vi "Fit Result to String.vi"(8 "error in (no error)":errorcluster, 11 "Abstract Fit in":refnum<class "Abstract Fit.lvclass">) -> (0 "error out":errorcluster, 2 "Array":string[](array[string]), 3 "Abstract Fit out":refnum<class "Abstract Fit.lvclass">)   [LabVIEW 2016, in "Abstract Fit.lvclass"]
uses:
  Abstract Fit.lvclass
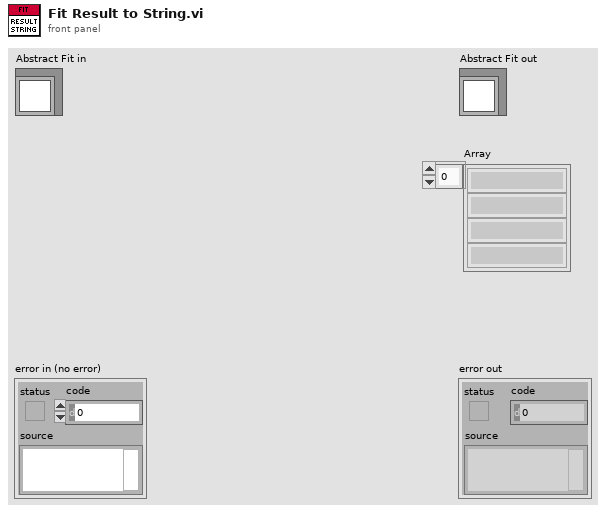
[diagram p1: front panel]
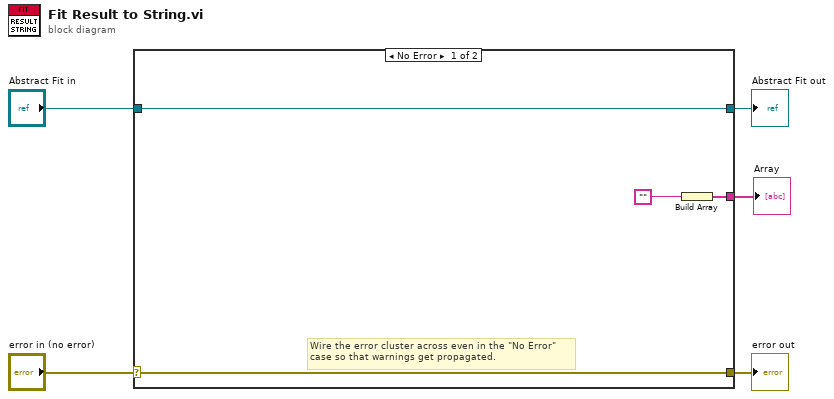
[diagram p0: block diagram]
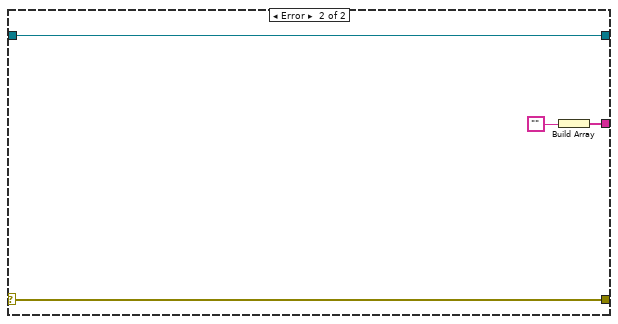
[diagram p2: hidden frame]
diagram:
  n1 = case shown="No Error" "error in (no error)" {
    selector: "error in (no error)" -> [w8 w13]
    tunnel: [w8 w13] -> w4
    tunnel: [w9 w12] -> w2
    tunnel: "Abstract Fit in" -> [w9 w12]
    tunnel: [w7 w10] -> w1
    frame No Error {
      # "Wire the error cluster across even in the \"No Error\"\ncase so that warnings get propagated."
      n2 = Build Array("") -> (w7:string[])
    }
    frame Error {
      n3 = Build Array("") -> (w10:string[])
    }
  }
  "error out" <- w4
  "Abstract Fit out" <- w2
  "Array" <- w1
